vi "Read roles.vi"(8 "error in (no error)":errorcluster, 11 "PreparePenaltyEnemyPlay in":refnum<class "PreparePenaltyEnemyPlay.lvclass">) -> (0 "error out":errorcluster, 2 "roles":T1, 3 "PreparePenaltyEnemyPlay out":refnum<class "PreparePenaltyEnemyPlay.lvclass">)   [LabVIEW 2020, in "PreparePenaltyEnemyPlay.lvclass"]
uses:
  PreparePenaltyEnemyPlay.lvclass
  PenaltyDefenseRole_class/PenaltyDefenseRole.lvclass
  PreparePenaltyEnemyPlay.lvclass/PreparePenaltyEnemyPlay.ctl
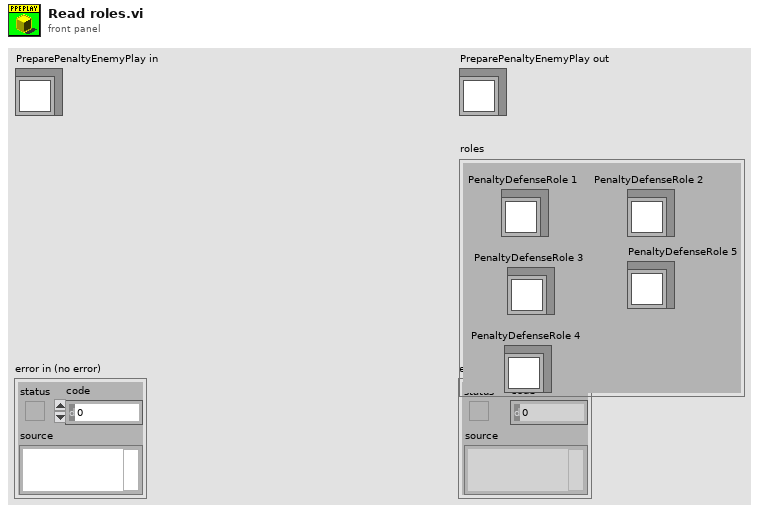
[diagram p1: front panel]
types:
  T1 = cluster{"PenaltyDefenseRole 1":refnum<class "PenaltyDefenseRole.lvclass">, "PenaltyDefenseRole 2":refnum<class "PenaltyDefenseRole.lvclass">, "PenaltyDefenseRole 3":refnum<class "PenaltyDefenseRole.lvclass">, "PenaltyDefenseRole 4":refnum<class "PenaltyDefenseRole.lvclass">, "PenaltyDefenseRole 5":refnum<class "PenaltyDefenseRole.lvclass">}
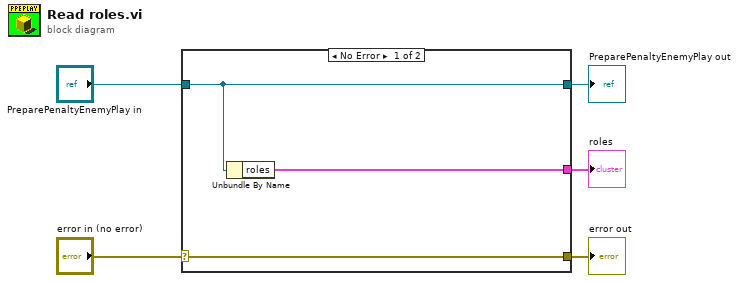
[diagram p0: block diagram]
diagram:
  n1 = case shown="No Error" "error in (no error)" {
    selector: "error in (no error)" -> [w8 w9]
    tunnel: [w8 w9] -> w4
    tunnel: [w7 w10] -> w2
    tunnel: "PreparePenaltyEnemyPlay in" -> [w7 w10]
    tunnel: [w6 _] -> w1
    frame No Error {
      n2 = Unbundle By Name(w7) -> ("roles"=w6:T1)
    }
    frame Error {
    }
  }
  "error out" <- w4
  "PreparePenaltyEnemyPlay out" <- w2
  "roles" <- w1
